vi "spectrum_fft.vi"() -> ()   [LabVIEW 2022 SP3]
uses:
  <vilib>/Analysis/4window.llb/windowTd.ctl
  <vilib>/Analysis/2dsp.llb/Real FFT.vi
  <vilib>/Analysis/0measdsp.llb/Scaled Time Domain Window (DBL).vi
  <vilib>/express/express analysis/Spectral/Block/exnSpectralBlock spectral measurements peak poly.vi
  <vilib>/express/express analysis/Spectral/Block/exnSpectralBlock spectral measurements peak DDT.vi
  <vilib>/express/express analysis/Spectral/XNode/ExpressSpectralMeasurementsBlockNode.xnode
  <vilib>/Analysis/NI_AALPro.lvlib
panel:
  in  "window":T1 items=["Rectangle"=0, "Hanning"=1, "Hamming"=2, "Blackman-Harris"=3, "Exact Blackman"=4, "Blackman"=5, "Flat Top"=6, "4 Term B-Harris "=7, "7 Term B-Harris"=8, "Low Sidelobe"=9, "Blackman Nuttall"=11, "Triangle"=30, "Bartlett-Hanning"=31, "Bohman"=32, "Parzen"=33, "Welch"=34, "Kaiser"=60, "Dolph-Chebyshev"=61, "Gaussian"=62]
  out "Waveform Graph 3":dbl[](graph)
  out "Waveform Graph 2":dbl[][](graph)
  out "Waveform Graph":dynamicdata(graph)
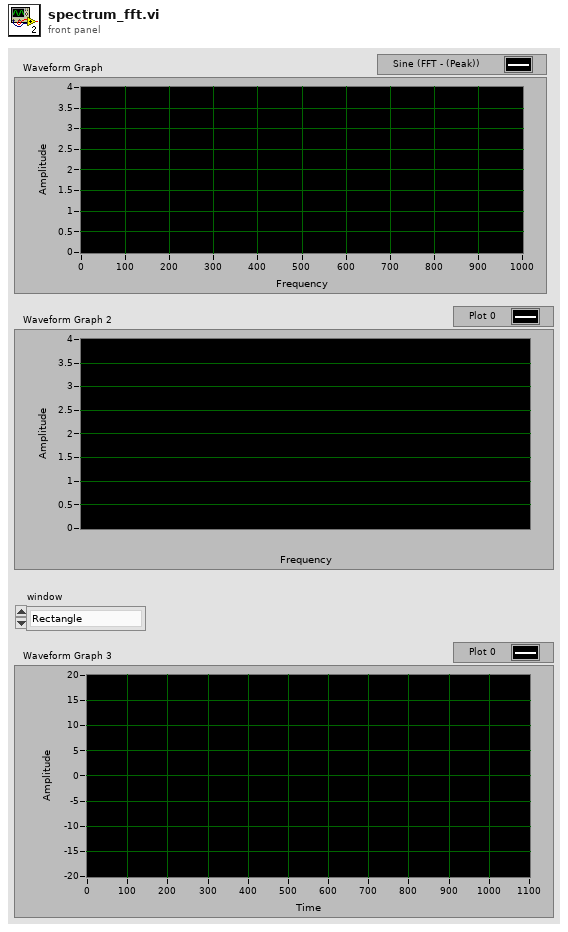
[diagram p1: front panel]
types:
  T1 = typedef "NI_AALPro.lvlib/windowTd.ctl" = u32
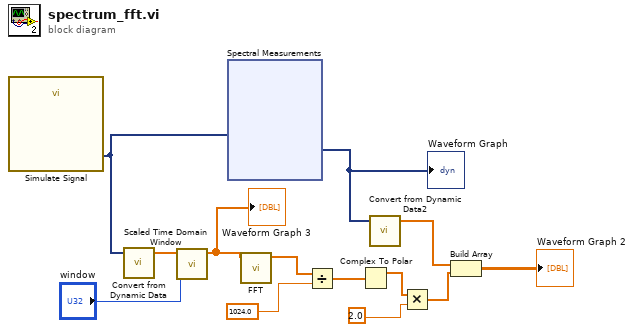
[diagram p0: block diagram]
diagram:
  n1 = call "Simulate Signal"() -> ("Sine"=w13:dynamicdata)  [unwired: 14 in, 1 out]
  n2 = call "Convert from Dynamic Data"("Dynamic Data Type"=w13) -> ("Array"=w2:dbl[])  [unwired: 3 in]
  n3 = call-poly <vilib>:"Scaled Time Domain Window.vi"("window"="window", "X"=w2) -> ("Windowed X"=w1:dbl[])  [unwired: 7 in, 2 out]
  "Waveform Graph 3" <- w1
  n4 = xnode "Spectral Measurements"("Signals"=w13) -> ("FFT - (Peak)"=w9:dynamicdata)  [unwired: 1 in, 2 out]
  "Waveform Graph" <- w9
  n5 = call-poly <vilib>:"FFT.vi"("X"=w1) -> ("FFT {X}"=w12:cdb[])  [unwired: 9 in, 1 out]
  n6 = Divide(x=w12, y=1024.0) -> (x/y=w10:cdb[])
  n7 = Complex To Polar(r * e^(i*theta)=w10) -> (r=w6:dbl[])  [unwired: 1 out]
  n8 = call "Convert from Dynamic Data2"("Dynamic Data Type"=w9) -> ("Array"=w8:dbl[])  [unwired: 3 in]
  n9 = Multiply(x=w6, y=2.0) -> (x*y=w4:dbl[])
  n10 = Build Array(w8, w4) -> (→"Waveform Graph 2":dbl[][])
